vi "Emballage_BDD_Lire  commandes GPAO.vi"(8 "error in":errorcluster, 9 "article":string="12-216C-04521 EQIFIL 104mA 230ohm", 10 "Numéro commande":string) -> (0 "error out":errorcluster, 1 "existe ?":bool=TRUE, 2 "Erreur de\n comunication":bool, 3 "Tab cmde GPAO":string[][](array[string])=[["12-216C-04521", "EQIFIL ", "104mA    230ohm", "03104/08-05.01.01", "3", "221769", "EMAIL VOM 01.04.08  ", "BLATTY AG", "", "      ", "Fluid Automation Systems SA             ", "ALL", "0"], ["12-216C-04521", "EQIFIL ", "104mA    230ohm", "03128/08-01.01.01", "2", "226006", "RETURN FROM VIASYS2 ", "Fluid Automat. Systems GmbH", "", "      ", "Fluid Automation Systems SA             ", "ALL", "1"], ["12-216C-04521", "EQIFIL ", "104mA    230ohm", "03130/08-01.01.01", "1", "226005", "RETURN FROM VIASYS1 ", "Fluid Automat. Systems GmbH", "", "      ", "Fluid Automation Systems SA             ", "ALL", "1"], ["12-216C-04521", "EQIFIL ", "104mA    230ohm", "03365/08-01.01.01", "4", "225536", "SANS PAPIERS GE     ", "Fluid Automat. Systems GmbH", "", "      ", "Fluid Automation Systems SA             ", "ALL", "1"], ["12-216C-04521", "EQIFIL ", "104mA    230ohm", "03570/08-02.01.01", "100", "225052", "SANS PAPIERS        ", "IMI International Sp. z o.o.", "", "      ", "Fluid Automation Systems SA             ", "ANG", "1"], ["12-216C-04521", "EQIFIL ", "104mA    230ohm", "05066/08-01.01.01", "13", "225726", "120830              ", "Fluid Automat. Systems GmbH", "", "      ", "Fluid Automation Systems SA             ", "ALL", "1"], ["12-216C-04521", "EQIFIL ", "104mA    230ohm", "05067/08-01.01.01", "11", "225727", "120831              ", "Fluid Automat. Systems GmbH", "", "      ", "Fluid Automation Systems SA             ", "ALL", "1"]], 4 "Indice REV":string, 5 "DATA cmde":T1={"n°article FAS"="12-216E-01-25 F120023 500mA 10ohm", "n° cmde FAS"="R03844/08-01.01.01", "quantité cmde"="4", "ID LIG cmde"="225540", "n° cmde client"="120565              ", "nom client"="Fluid Automat. Systems GmbH", "n° article client"="21088", "indice revision client"="      ", "société de facturation"="FAS Medic SA                            ", "langue a utiliser"="ALL"})   [LabVIEW 2020]
doc: "Liste les commandes relatives au produit à emballer dans la GPAO.\nRenvoie un tableau contenant :\n 0 - le n° article FAS (ex. 12-216C-04520)\n 1 - le n° FILE FAS (ex. F120023)\n 2 - la designation du produit (ex. 211mA 57ohm)\n 3 - le n° cmde FAS\n 4 - la quantité à emballer\n 5 - ID cmde\n 6 - le n° cmde client\n 7 - le nom du client\n 8 - n° article client\n 9 - indice revision client\n 10 - société de facturation\n 11 - langue à utiliser\n 12 - retour? 0 non, 1 oui"
uses:
  Modules/FS/60_FS_Controles/60_FS_SetGet.ctl
  <vilib>/addons/database/Connection.llb/DB Tools Open Connec (Path).vi
  <vilib>/addons/database/NI_Database_API.lvlib
panel:
  out "temps Exe [s]":dbl
  in  "Indication commande non facturée":string="and (CDE_FACTURE=0)"
  out "requete":string="where (NO_ARTICLE ='12-216C-04521') and (NO_FILE ='EQIFIL') and (DESIGNATION LIKE '%104mA%')"
  in  "requete manuelle":string="where (NO_FILE='F120054')"
  in  "columns com":string[](array[string])=["NO_ARTICLE", "NO_FILE", "DESIGNATION", "NO_CDEVAL", "QUANTITE_VAL", "DATE_LIV_PREV", "ID_LIG_CDE_VAL", "REF_COMMANDE_CLT", "NOM_CLIENT", "REF_ARTICLE_CLIENT", "INDICE_REVISION_CLT", "SOC_FACTURATION", "LANGUE", "QUANTITE_DEM", "RETOUR_CLIENT", "INDICE_REV", "ID_ARTICLE"]
  in  "Table com":string="V_P_LIGCDEVAL"
  # "01-211E-01-H6 F011013 18V DC 4,5W\tMK0228506AR\tAMIIII\t20\tCDA\tn\to\n01-211E-01-H6 F011014 18V DC 4,5W\tMK0228606AR\tAMIIII\t20\tCDA\tn\to\n01-211P-03-26 F011129 5_1,5V DC 4,2_0,4W\tM3566503AR\tAMIIII\t20\tCDA\tn\to\n04-341E-11-11 F04313 4212 SDGNUL 24V DC 10W\t860262411AR\tAMIIII\t4\tCDA\tn\to\n01-223E-01-B6 F011107 18V DC 4,5W\tMK0185209AR\tAMIIII\t20\tCDA\tn\to\n01-211E-01-H6 F01938 18V DC 4,5W\tMK0185009AR\tAMIIII\t20\tCDA\tn\to\n01-213E-01-B6 F011106 18V DC 4,5W\tMK0185109AR\tAMIIII\t20\tCDA\tn\to\nS002.0002 BLOC 2P TRILOGY\t0002000203\tAASSIIII\t4\tCDA\tn\to\n04-331E-11-11 F040340 258 SDGNUL 24V DC 14,5W\tMK0158508AR\tAMIIII\t5\tCDA\tn\to\n04-341E-11-11 F040376 4212 SDGNUL 24V DC 10W\tMK0354102AR\tAMIIII\t4\tCDA\tn\to\n04-341E-11-11 F040408 4212 BFLSDG 24V DC 10W\t860202410AR\tAMIIII\t4\tCDA\tn\to\nS122.0071 CARINA AVEC FILTRE FERRITE\t570497500SR\tAMIIII\t24\tCDA\tn\to\nS122.0009 BLOC DAGMAR DIGITAL\tMK0206008AR\tAMIIII\t1\tCDA\tn\to\nS112.1289 BLOC 3P CALIBRATION UNIT\t841521316AR\tAMIIII\t24\tCDA\tn\to\nS012.1247 GASEINGANGSBLOCK 8411848\t8411848-12AR\tAM-IIII\t1\tCDA\tn\to\nS122.0008 DOSIERPATRONE (AUSTAUSCH-SET)\tMK0205706AR\tAMIIII\t1\tCDA\tn\to"
  # "12-216E-01-25 F120023 500mA 10Ohm"
  # "12-216C-04521 F120073 211mA 57ohm"
  # "where (NO_ARTICLE ='17-216C-00341') and (NO_FILE ='D3WFIL') and (DESIGNATION LIKE '% 42mA%')and (CDE_FACTURE=0)"
  # "12-216C-04520 EQIFIL 211mA 57ohm"
  # "12-216C-01-41 F120044 264mA 36ohm"
  # "12-216C-04521 EQIFIL 417mA 14.4ohm"
  # "0"
  # "12-216C-01-41"
  # "1"
  # "F120044"
  # "2"
  # "264mA     36ohm"
  # "03063/08-02.01.02"
  # "3"
  # "4"
  # "qtté à emballer"
  # "0 => non facturée\n1 => facturée\nsans cette requette => additionne les deux types de commande"
  # "5"
  # "6"
  # "7"
  # "8"
  # "9"
  # "10"
  # "11"
  # "FAS Medic SA/Fluid Automation Systems SA"
  # "12"
  # "ANG/FR/ALL/E/I"
  # "13"
  # "qtté totale"
  # "0 normal ; 1 retour"
  # "14"
  # "15"
  # "Indice Rev"
  # "16"
  # "7"
  # "8"
  # "9"
  # "10"
  # "0"
  # "1"
  # "2"
  # "3"
  # "4"
  # "11"
  # "12"
  # "14"
  # "15"
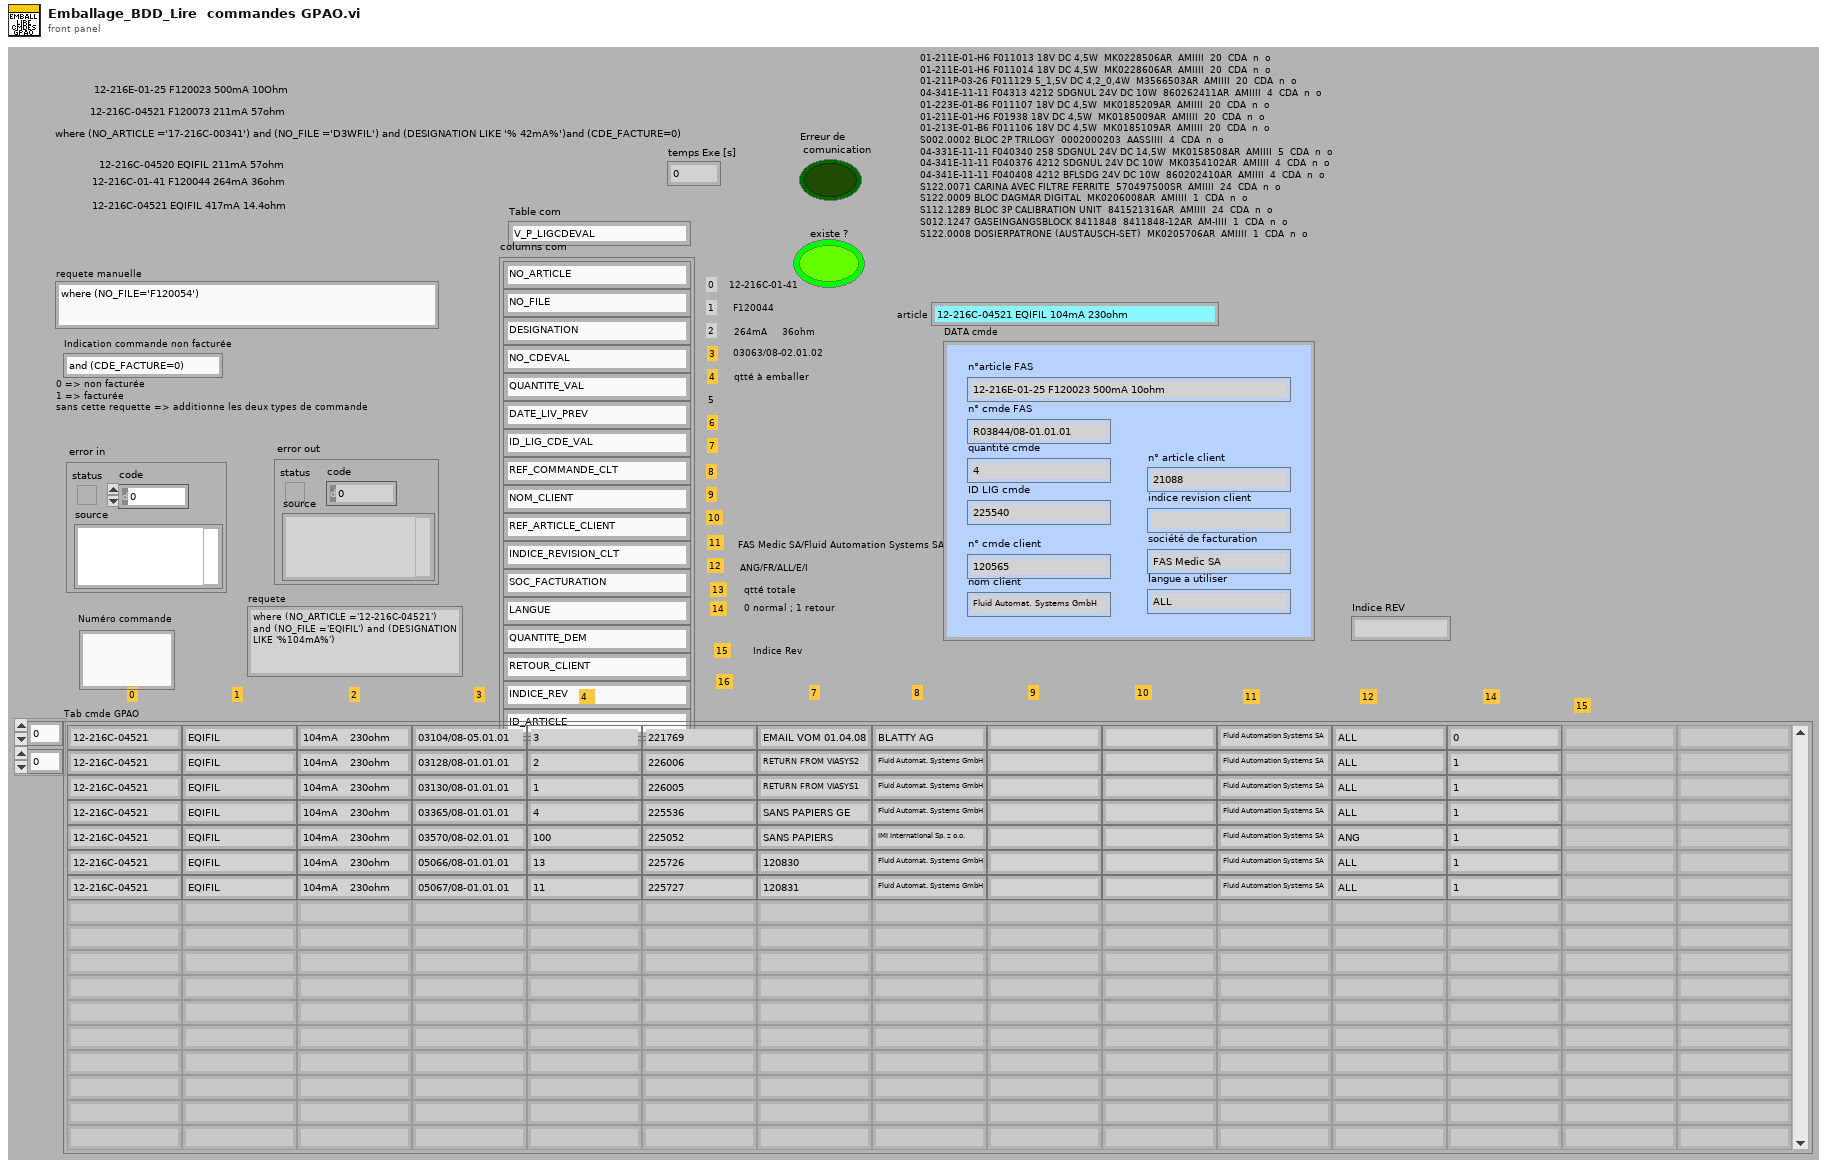
[diagram p1: front panel]
types:
  T1 = typedef "DATA commande.ctl" = cluster{"n°article FAS":string, "n° cmde FAS":string, "quantité cmde":string, "ID LIG cmde":string, "n° cmde client":string, "nom client":string, "n° article client":string, "indice revision client":string, "société de facturation":string, "langue a utiliser":string}
  T2 = typedef "60_FS_SetGet.ctl" = enum16{"set", "get"}
  T3 = typedef "60_FS_CLT_Chemins.ctl" = cluster{"Racine_local":path, "Racine_reseau":path, "Racine_Support_Application":path, "Fichier_Journalisation":path, "Connexion_BDD_VSX":path, "Connexion_BDD_PLZ":path}
  T4 = typedef "NI_Database_API.lvlib/Conn ObjectReference.ctl" = refnum<k1>
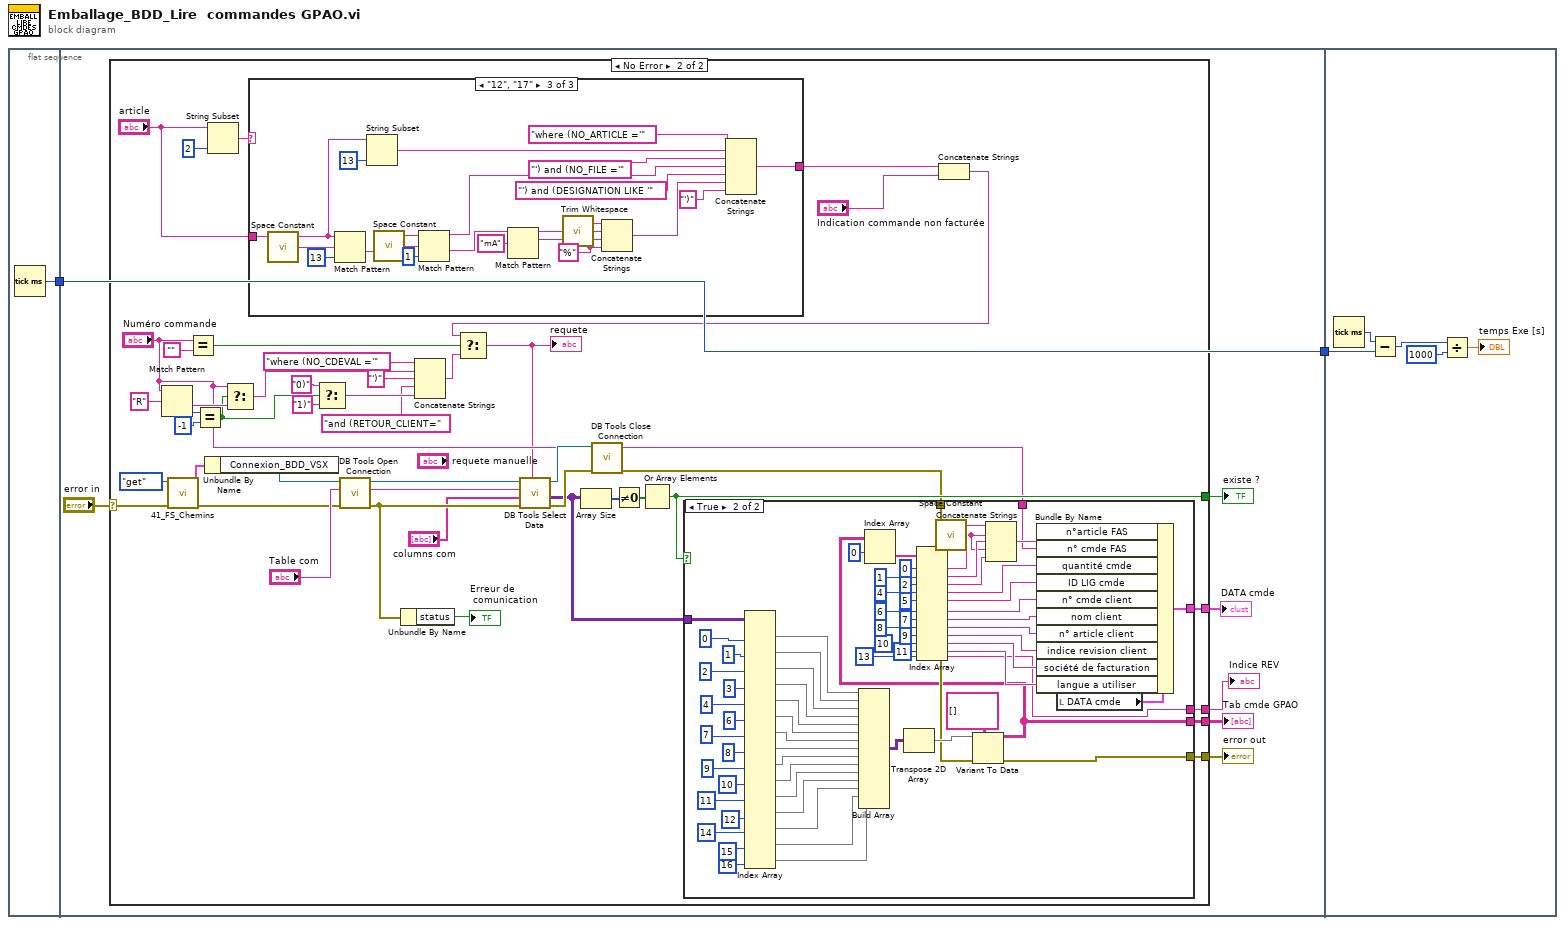
[diagram p0: block diagram]
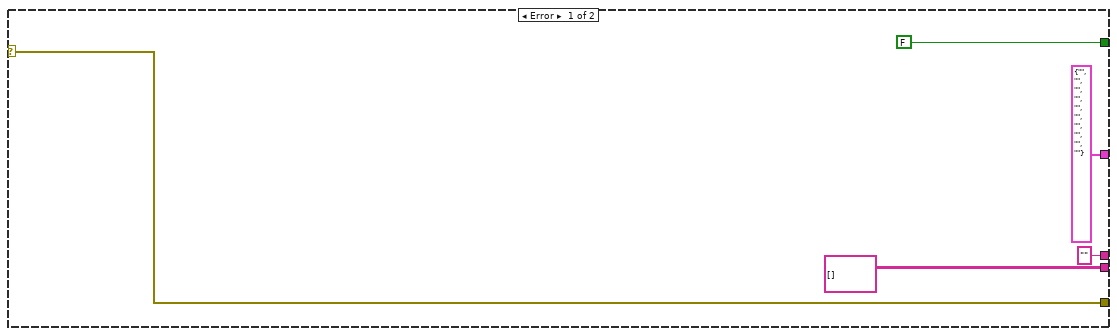
[diagram p2: hidden frame]
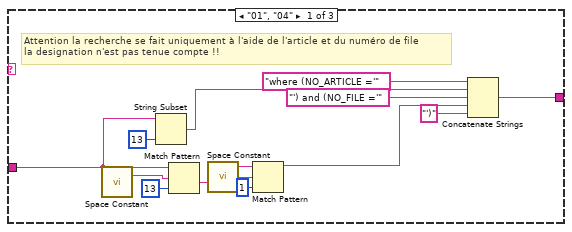
[diagram p3: hidden frame]
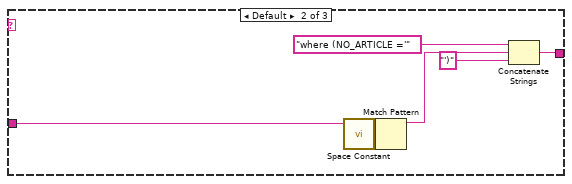
[diagram p4: hidden frame]
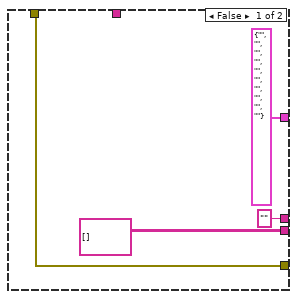
[diagram p5: hidden frame]
diagram:
  n1 = flat-sequence {
    tunnel: [w3] -> w1
    tunnel: [w5] -> w2
    tunnel: w1 -> [w5]
    tunnel: w2 -> [w172]
    frame #0 {
      n2 = Tick Count (ms)() -> (millisecond timer value=w3:u32)
    }
    frame #1 {
      n3 = case shown="No Error" "error in" {
        selector: "error in" -> [w14 w20]
        tunnel: [w14 w52] -> w10
        tunnel: [FALSE w55] -> w8
        tunnel: [string[][] [] w50] -> w7
        tunnel: [T1 {"n°article FAS"="", "n° cmde FAS"="", "quantité cmde"="", "ID LIG cmde"="", "n° cmde client"="", "nom client"="", "n° article client"="", "indice revision client"="", "société de facturation"="", "langue a utiliser"=""} ("DATA cmde") w27] -> w6
        tunnel: ["" ("DATE_EMBALLAGE") w17] -> w4
        frame Error {
        }
        frame No Error {
          n4 = Match Pattern(string="Numéro commande", regular expression="R" ("expression régulière")) -> (after substring=w35:string, offset past match=w37:i32)  [unwired: 1 in, 2 out]
          n5 = call "41_FS_Chemins.vi"("error in (no error)"=w20, "SetGet"=60_FS_SetGet."get") -> ("error out"=w19:errorcluster, "CLT_Chemins_out"=w22:T3)  [unwired: 8 in]
          n6 = Equal?(x="Numéro commande", y="") -> (x = y?=w45:bool)
          n7 = Equal?(x=w37, y=-1) -> (x = y?=w33:bool)
          n8 = Unbundle By Name(w22) -> ("Connexion_BDD_VSX"=w18:path)
          n9 = String Subset(string="article", length (rest)=2 ("longueur (reste)")) -> (substring=w48:string)  [unwired: 1 in]
          n10 = Select(t="Numéro commande", s=w33, f=w35) -> (s? t:f=w34:string)
          n11 = case shown="\"12\", \"17\"" w48 {
            tunnel: "article" -> [w69 w74 w89]
            tunnel: [w72 w76 w86] -> w41
            frame "01", "04" {
              # "Attention la recherche se fait uniquement à l'aide de l'article et du numéro de file\nla designation n'est pas tenue compte !!"
              n12 = call <vilib>:"Space Constant.vi"() -> ("String"=w65:string)
              n13 = String Subset(string=w69, length (rest)=13 ("longueur (reste)")) -> (substring=w70:string)  [unwired: 1 in]
              n14 = Match Pattern(string=w69, regular expression=w65, offset (0)=13) -> (after substring=w67:string)  [unwired: 3 out]
              n15 = call <vilib>:"Space Constant.vi"() -> ("String"=w66:string)
              n16 = Match Pattern(string=w67, regular expression=w66, offset (0)=1) -> (before substring=w71:string)  [unwired: 3 out]
              n17 = Concatenate Strings("where (NO_ARTICLE ='" ("optional clause"), w70, "') and (NO_FILE ='" ("chaîne"), w71, "')" ("chaîne")) -> (w72:string)
            }
            frame Default {
              n18 = call <vilib>:"Space Constant.vi"() -> ("String"=w75:string)
              n19 = Match Pattern(string=w74, regular expression=w75) -> (before substring=w73:string)  [unwired: 1 in, 3 out]
              n20 = Concatenate Strings("where (NO_ARTICLE ='" ("optional clause"), w73, "')" ("chaîne")) -> (w76:string)
            }
            frame "12", "17" {
              w81 = "%" ("chaîne")
              n21 = call <vilib>:"Space Constant.vi"() -> ("String"=w92:string)
              n22 = Match Pattern(string=w89, regular expression=w92, offset (0)=13) -> (after substring=w94:string)  [unwired: 3 out]
              n23 = String Subset(string=w89, length (rest)=13 ("longueur (reste)")) -> (substring=w88:string)  [unwired: 1 in]
              n24 = call <vilib>:"Space Constant.vi"() -> ("String"=w93:string)
              n25 = Match Pattern(string=w94, regular expression=w93, offset (0)=1) -> (before substring=w87:string, after substring=w85:string)  [unwired: 2 out]
              n26 = Match Pattern(string=w85, regular expression="mA") -> (before substring=w80:string, match substring=w83:string)  [unwired: 1 in, 2 out]
              n27 = call <vilib>:"Trim Whitespace.vi"("string"=w80) -> ("trimmed string"=w79:string)  [unwired: 1 in]
              n28 = Concatenate Strings(w81, w79, w83, w81) -> (w82:string)
              n29 = Concatenate Strings("where (NO_ARTICLE ='" ("optional clause"), w88, "') and (NO_FILE ='" ("chaîne"), w87, "') and (DESIGNATION LIKE '" ("chaîne"), w82, "')" ("chaîne")) -> (w86:string)
            }
          }
          n30 = Select(t="0)", s=w33, f="1)") -> (s? t:f=w32:string)
          n31 = call-poly <vilib>:"DB Tools Open Connection.vi"("error in (no error)"=w19, "connection information"=w18) -> ("error out"=w24:errorcluster, "connection reference"=w26:T4)  [unwired: 6 in]
          n32 = Unbundle By Name(w24) -> ("status"=→"Erreur de\n comunication":bool)
          n33 = Concatenate Strings("where (NO_CDEVAL ='" ("chaîne"), w34, "')" ("chaîne"), "and (RETOUR_CLIENT=" ("cas faux"), w32) -> (w42:string)
          n34 = Concatenate Strings(w41, "Indication commande non facturée") -> (w40:string)
          n35 = Select(t=w40, s=w45, f=w42) -> (s? t:f=w16:string)
          "requete" <- w16
          n36 = call <vilib>:"DB Tools Select Data.vi"("condition"=w16, "error in (no error)"=w24, "columns"="columns com", "table"="Table com", "connection reference"=w26) -> ("error out"=w57:errorcluster, "data"=w51:variant[][], "connection reference out"=w56:T4)  [unwired: 1 in]
          n37 = Array Size(array=w51) -> (size(s)=w59:i32[])
          n38 = call <vilib>:"DB Tools Close Connection.vi"("error in (no error)"=w57, "connection reference"=w56) -> ("error out"=w54:errorcluster)  [unwired: 5 in]
          n39 = Not Equal To 0?(x=w59) -> (x != 0?=w58:bool[])
          n40 = Or Array Elements(Boolean array=w58) -> (logical OR=w55:bool)
          n41 = case shown="True" w55 {
            tunnel: w51 -> [_ w165]
            tunnel: w54 -> [w103 w163]
            tunnel: [w103 w149] -> w52
            tunnel: [string[][] [] w113] -> w50
            tunnel: "Numéro commande" -> [_ w112]
            tunnel: [T1 {"n°article FAS"="", "n° cmde FAS"="", "quantité cmde"="", "ID LIG cmde"="", "n° cmde client"="", "nom client"="", "n° article client"="", "indice revision client"="", "société de facturation"="", "langue a utiliser"=""} ("DATA cmde") w110] -> w27
            tunnel: ["" ("DATE_EMBALLAGE") w106] -> w17
            frame False {
            }
            frame True {
              n42 = Index Array(array=w165, index (col) #1=0 ("indice désactivé (col)"), index (col) #2=1 ("indice désactivé (col)"), index (col) #3=2 ("indice désactivé (col)"), index (col) #4=3 ("indice désactivé (col)"), index (col) #5=4 ("indice désactivé (col)"), index (col) #6=6 ("indice désactivé (col)"), index (col) #7=7 ("indice désactivé (col)"), index (col) #8=8 ("indice désactivé (col)"), index (col) #9=9 ("indice désactivé (col)"), index (col) #10=10 ("indice désactivé (col)"), index (col) #11=11 ("indice désactivé (col)"), index (col) #12=12 ("indice désactivé (col)"), index (col) #13=14 ("indice désactivé (col)"), index (col) #14=15 ("indice désactivé (col)"), index (col) #15=16 ("indice (col)")) -> (element #1=w142:variant[], element #2=w143:variant[], element #3=w144:variant[], element #4=w167:variant[], element #5=w157:variant[], element #6=w156:variant[], element #7=w155:variant[], element #8=w154:variant[], element #9=w153:variant[], element #10=w152:variant[], element #11=w151:variant[], element #12=w150:variant[], element #13=w140:variant[], element #14=w108:variant[], element #15=w104:variant[])  [unwired: 15 in]
              n43 = Build Array(w142, w143, w144, w167, w157, w156, w155, w154, w153, w152, w151, w150, w140, w108, w104) -> (w168:variant[][])
              n44 = Transpose 2D Array(2D array=w168) -> (transposed array=w169:variant[][])
              n45 = call <vilib>:"Space Constant.vi"() -> ("String"=w111:string)
              n46 = Variant To Data(error in=w163, type=string[][] [], Variant=w169) -> (data=w113:string[][], error out=w149:errorcluster)
              n47 = Index Array(array=w113, index (row)=0 ("indice (ligne)")) -> (element=w114:string[])  [unwired: 1 in]
              n48 = Index Array(array=w114, index #1=0 ("indice"), index #2=1 ("indice"), index #3=2 ("indice"), index #4=4 ("indice"), index #5=5 ("indice"), index #6=6 ("indice"), index #7=7 ("indice"), index #8=8 ("indice"), index #9=9 ("indice"), index #10=10 ("indice"), index #11=11 ("indice"), index #12=13 ("indice")) -> (element #1=w125:string, element #2=w126:string, element #3=w127:string, element #4=w128:string, element #5=w129:string, element #6=w130:string, element #7=w131:string, element #8=w132:string, element #9=w133:string, element #10=w135:string, element #11=w137:string, element #12=w106:string)
              n49 = Concatenate Strings(w125, w111, w126, w111, w127) -> (w124:string)
              n50 = local read "DATA cmde"() -> (w139:T1)
              n51 = Bundle By Name(cluster=w139, "n°article FAS"=w124, "n° cmde FAS"=w112, "quantité cmde"=w128, "ID LIG cmde"=w129, "n° cmde client"=w130, "nom client"=w131, "n° article client"=w132, "indice revision client"=w133, "société de facturation"=w135, "langue a utiliser"=w137) -> (w110:T1)
            }
          }
        }
      }
      "error out" <- w10
      "existe ?" <- w8
      "Tab cmde GPAO" <- w7
      "DATA cmde" <- w6
      "Indice REV" <- w4
    }
    frame #2 {
      n52 = Tick Count (ms)() -> (millisecond timer value=w176:u32)
      n53 = Subtract(x=w176, y=w172) -> (x-y=w173:u32)
      n54 = Divide(x=w173, y=u32 1000) -> (x/y=→"temps Exe [s]":dbl)
    }
  }
